vi "Write Ignore Array.vi"(8 "error in (no error)":errorcluster, 10 "IgnoreArr":bool, 11 "IntensityChart.lvclass in":refnum<class "IntensityChart.lvclass">) -> (0 "error out":errorcluster, 3 "IntensityChart.lvclass out":refnum<class "IntensityChart.lvclass">)   [LabVIEW 2015, in "IntensityChart.lvclass"]
uses:
  IntensityChart.lvclass
  IntensityChart.lvclass/IntensityChart.ctl
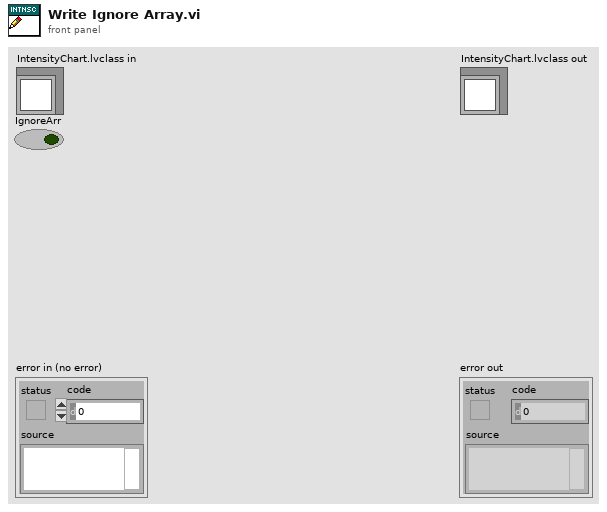
[diagram p1: front panel]
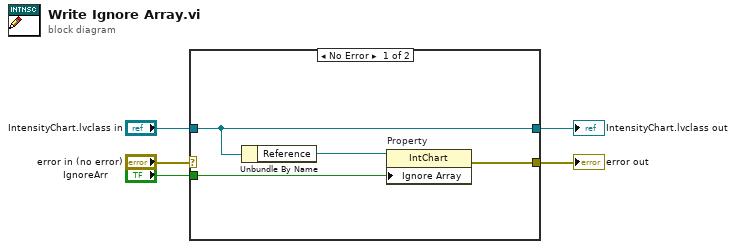
[diagram p0: block diagram]
diagram:
  n1 = case shown="No Error" "error in (no error)" {
    selector: "error in (no error)" -> [_ w11]
    tunnel: [w9 w11] -> w4
    tunnel: [w7 w10] -> w2
    tunnel: "IntensityChart.lvclass in" -> [w7 w10]
    tunnel: "IgnoreArr" -> [w8 _]
    frame No Error {
      n2 = Unbundle By Name(w7) -> ("Reference"=w6:refnum<vi>)
      n3 = property on="Property" class="IntChart"(reference=w6, "Ignore Array"=w8) -> (error out=w9:errorcluster)  [unwired: 1 in, 1 out]
    }
    frame Error {
    }
  }
  "error out" <- w4
  "IntensityChart.lvclass out" <- w2
